vi "Get Calibration from File.vi"(10 "Pump Calibration":u16, 11 "Pump Module Config":T1) -> (2 "Calibration Y Intercept":dbl, 3 "Calibration Slope":dbl)   [LabVIEW 2018, in "Centrifuge Module.lvlib"]
uses:
  Centrifuge Module.lvlib
  <vilib>/Utility/file.llb/Read Delimited Spreadsheet (string).vi
  <vilib>/Utility/miscctls.llb/LVPoint32TypeDef.ctl
  Centrifuge Module Settings Cluster.ctl
  Centrifuge Module Config Cluster.ctl
  EPOS4/EPOS Communication Serttings.ctl
  EPOS4/Device Selection.ctl
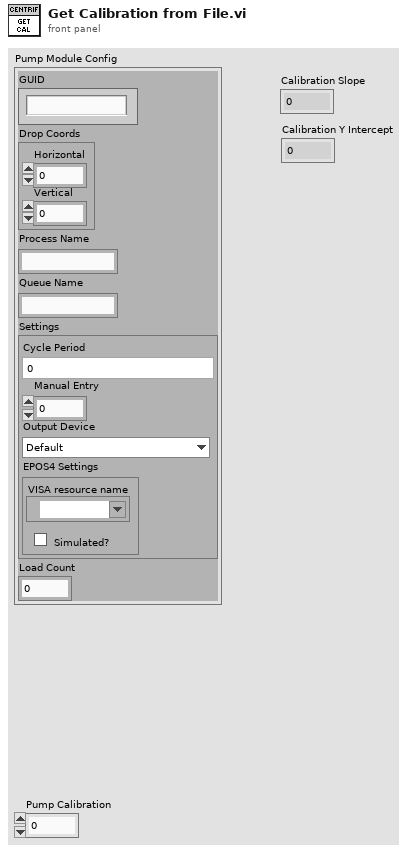
[diagram p1: front panel]
types:
  T1 = typedef "Centrifuge Module.lvlib/Centrifuge Module Config Cluster.ctl" = cluster{"GUID":string, "Drop Coords":T2, "Process Name":string, "Queue Name":string, "Settings":T3, "Load Count":i32}
  T2 = typedef "LVPoint32TypeDef.ctl" = cluster{"Horizontal":i32, "Vertical":i32}
  T3 = typedef "Centrifuge Module.lvlib/Centrifuge Module Settings Cluster.ctl" = cluster{"Cycle Period":dbl, "Manual Entry":dbl, "Output Device":T4, "EPOS4 Settings":T5}
  T4 = typedef "Device Selection.ctl" = enum16{"Default", "EPOS4"}
  T5 = typedef "EPOS Communication Serttings.ctl" = cluster{"VISA resource name":refnum<visa-resource-name>, "Simulated?":bool}
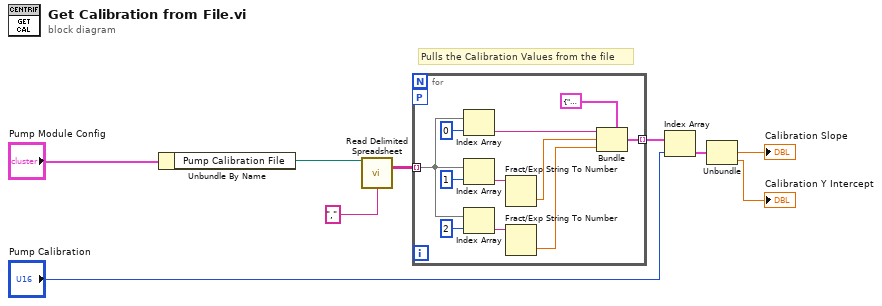
[diagram p0: block diagram]
diagram:
  # "Pulls the Calibration Values from the file"
  n1 = Unbundle By Name("Pump Module Config") -> ("Pump Calibration File"=w4:path)
  n2 = call-poly <vilib>:"Read Delimited Spreadsheet.vi"("file path (dialog if empty)"=w4, "delimiter (\\t)"="," ("delimiter (\\t)")) -> ("all rows"=w2:string[][])  [unwired: 8 in, 5 out]
  n3 = for {
    tunnel: w2 -> [w11] mode=indexing
    tunnel: [w15] -> w7 mode=indexing
    workers-P: _ -> [_]
    n4 = Index Array(array=w11, index=0) -> (element=w17:string)
    n5 = Index Array(array=w11, index=1) -> (element=w14:string)
    n6 = Index Array(array=w11, index=2) -> (element=w12:string)
    n7 = Fract/Exp String To Number(string=w14) -> (number=w18:dbl)  [unwired: 3 in, 1 out]
    n8 = Fract/Exp String To Number(string=w12) -> (number=w10:dbl)  [unwired: 3 in, 1 out]
    n9 = Bundle(cluster=cluster{"String":string, dbl, dbl} {"String"="", 0.0, 0.0}, "String"=w17, w18, w10) -> (w15:cluster{"String":string, dbl, dbl})
  }
  n10 = Index Array(array=w7, index="Pump Calibration") -> (element=w8:cluster{"String":string, dbl, dbl})
  n11 = Unbundle(w8) -> (→"Calibration Slope":dbl, →"Calibration Y Intercept":dbl)  [unwired: 1 out]
